vi "calculate.vi"(0 "wm":dbl, 1 "input_1":dbl, 2 "RefpropDirectory":string, 3 "n":i32, 5 "input_2":dbl, 7 "units":enum16{"SI", "IP"}(ring), 9 "InpCode":T1(ring), 11 "error in":errorcluster, 12 "x":dbl[](array[numeric]), 14 "Clear Memory":bool) -> (4 "dataout":dbl[](array[numeric]), 13 "files_path_out":path, 15 "error out":errorcluster)   [LabVIEW 2017]
doc: "Please feel free to contact me if you have any questions .\nMy mail:ken_pop@tom.com yan.ding@jci.com"
panel:
  out "memory counter":i32
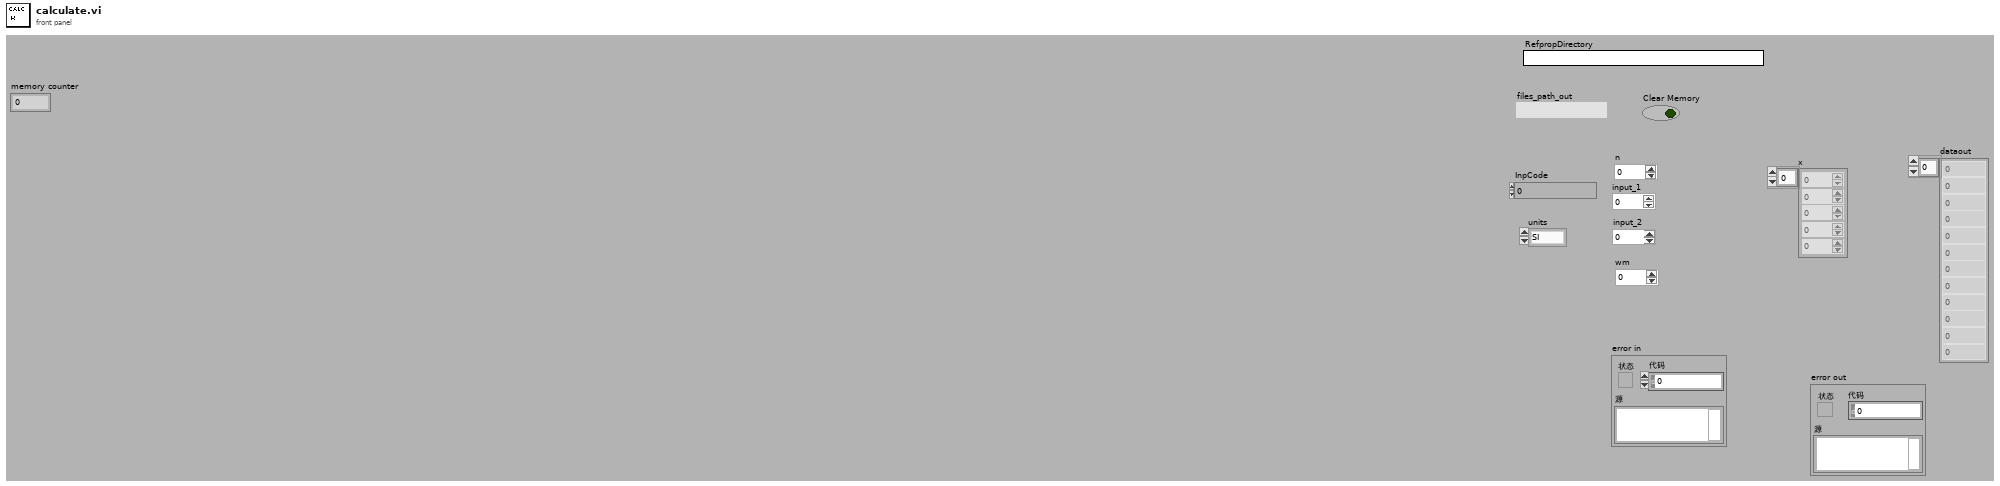
[diagram p1: front panel]
types:
  T1 = enum16{"0", "PS", "HS", "T", "P", "TP", "TH", "TS", "PH", "PQ", "TQ"}
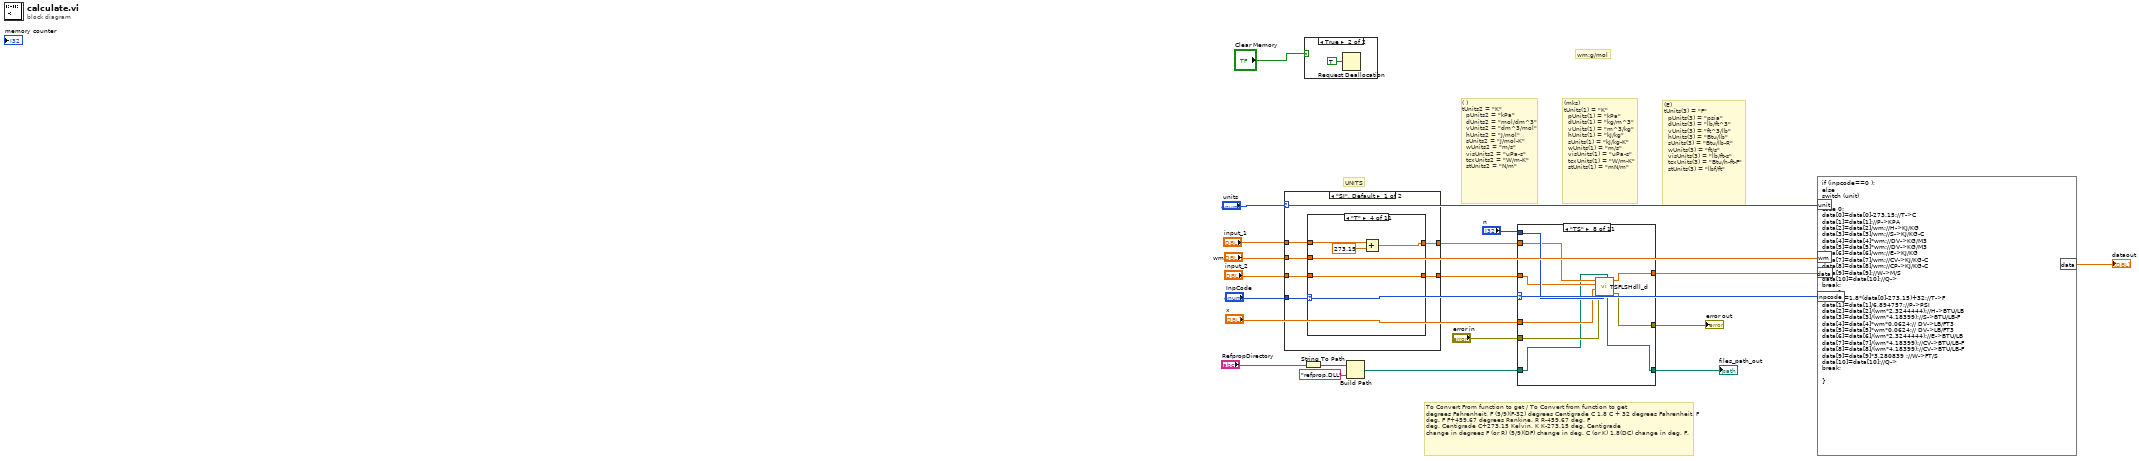
[diagram p0: block diagram]
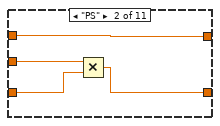
[diagram p4: hidden frame]
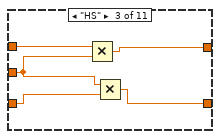
[diagram p5: hidden frame]
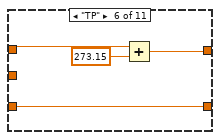
[diagram p7: hidden frame]
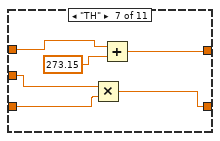
[diagram p8: hidden frame]
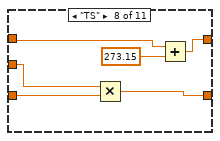
[diagram p9: hidden frame]
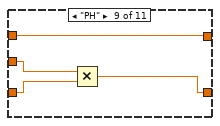
[diagram p10: hidden frame]
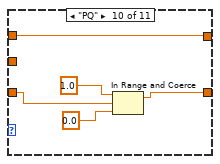
[diagram p11: hidden frame]
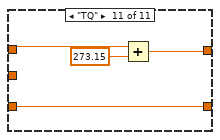
[diagram p12: hidden frame]
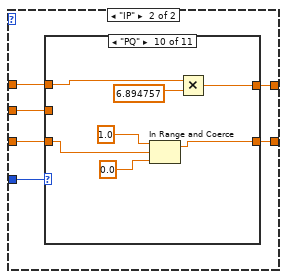
[diagram p13: hidden frame]
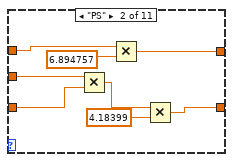
[diagram p15: hidden frame]
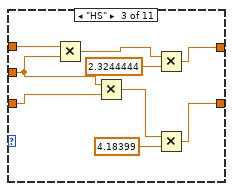
[diagram p16: hidden frame]
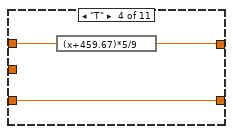
[diagram p17: hidden frame]
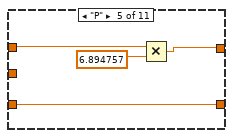
[diagram p18: hidden frame]
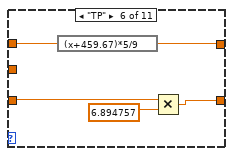
[diagram p19: hidden frame]
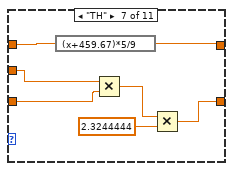
[diagram p20: hidden frame]
diagram:
  # "To Convert From function to get / To Convert from function to get \ndegrees Fahrenheit, F (5/9)(F-32) degrees Centigrade C 1.8 C + 32 degrees Fahrenheit, F \ndeg. F F+459.67 degrees Rankine, R R-459.67 deg. F \ndeg. Centigrade C+273.15 Kelvin, K K-273.15 deg. Centigrade \nchange in degrees F (or R) (5/9)(DF) change in deg. C (or K) 1.8(DC) change in deg. F."
  # "wm:g/mol"
  # "UNITS"
  # "(E)\ntUnits(3) = \"F\"\n  pUnits(3) = \"psia\"\n  dUnits(3) = \"lb/ft^3\"\n  vUnits(3) = \"ft^3/lb\"\n  hUnits(3) = \"Btu/lb\"\n  sUnits(3) = \"Btu/lb-R\"\n  wUnits(3) = \"ft/s\"\n  visUnits(3) = \"lb/ft-s\"\n  tcxUnits(3) = \"Btu/h-ft-F\"\n  stUnits(3) = \"lbf/ft\""
  # "(mks)\ntUnits(1) = \"K\"\n  pUnits(1) = \"kPa\"\n  dUnits(1) = \"kg/m^3\"\n  vUnits(1) = \"m^3/kg\"\n  hUnits(1) = \"kJ/kg\"\n  sUnits(1) = \"kJ/kg-K\"\n  wUnits(1) = \"m/s\"\n  visUnits(1) = \"uPa-s\"\n  tcxUnits(1) = \"W/m-K\"\n  stUnits(1) = \"mN/m\""
  # "( )\ntUnits2 = \"K\"\n  pUnits2 = \"kPa\"\n  dUnits2 = \"mol/dm^3\"\n  vUnits2 = \"dm^3/mol\"\n  hUnits2 = \"J/mol\"\n  sUnits2 = \"J/mol-K\"\n  wUnits2 = \"m/s\"\n  visUnits2 = \"uPa-s\"\n  tcxUnits2 = \"W/m-K\"\n  stUnits2 = \"N/m\""
  n1 = case shown="\"SI\", Default" "units" {
    tunnel: "InpCode" -> [w25 w72]
    tunnel: "input_1" -> [w24 w75]
    tunnel: [w23 w77] -> w9
    tunnel: "input_2" -> [w22 w73]
    tunnel: [w21 w76] -> w7
    tunnel: "wm" -> [w20 w74]
    frame "SI", Default {
      n2 = case shown="\"T\"" w25 {
        tunnel: w24 -> [w27 w31 w36 w39 w42 w45 w51 w57 w59 w65 w70]
        tunnel: [w27 w31 w32 w38 w42 w44 w50 w56 w59 w65 w69] -> w23
        tunnel: w22 -> [w26 w29 w34 w37 w41 w43 w48 w54 w61 w64 w68]
        tunnel: [w26 w28 w33 w37 w41 w43 w47 w53 w60 w63 w68] -> w21
        tunnel: w20 -> [_ w30 w35 _ _ _ w49 w55 w62 _ _]
        frame "0", Default {
        }
        frame "PS" {
          n3 = Multiply(x=w30, y=w29) -> (x*y=w28:dbl)
        }
        frame "HS" {
          n4 = Multiply(x=w36, y=w35) -> (x*y=w32:dbl)
          n5 = Multiply(x=w35, y=w34) -> (x*y=w33:dbl)
        }
        frame "T" {
          n6 = Add(x=w39, y=273.15) -> (x+y=w38:dbl)
        }
        frame "P" {
        }
        frame "TP" {
          n7 = Add(x=w45, y=273.15) -> (x+y=w44:dbl)
        }
        frame "TH" {
          n8 = Multiply(x=w49, y=w48) -> (x*y=w47:dbl)
          n9 = Add(x=w51, y=273.15) -> (x+y=w50:dbl)
        }
        frame "TS" {
          n10 = Multiply(x=w55, y=w54) -> (x*y=w53:dbl)
          n11 = Add(x=w57, y=273.15) -> (x+y=w56:dbl)
        }
        frame "PH" {
          n12 = Multiply(x=w62, y=w61) -> (x*y=w60:dbl)
        }
        frame "PQ" {
          n13 = In Range and Coerce(upper limit=1.0 ("上限"), x=w64, lower limit=0.0 ("下限")) -> (coerced(x)=w63:dbl)  [unwired: 1 out]
        }
        frame "TQ" {
          n14 = Add(x=w70, y=273.15) -> (x+y=w69:dbl)
        }
      }
    }
    frame "IP" {
      n15 = case shown="\"PQ\"" w72 {
        tunnel: w75 -> [w79 w84 w96 w98 w101 w105 w110 w117 w127 w132 w140]
        tunnel: [w79 w83 w88 w97 w100 w104 w109 w116 w126 w131 w139] -> w77
        tunnel: w73 -> [w78 w86 w94 w99 w103 w107 w114 w121 w129 w135 w138]
        tunnel: [w78 w80 w91 w99 w103 w106 w111 w118 w123 w134 w138] -> w76
        tunnel: w74 -> [_ w87 w95 _ _ _ w115 w122 w130 _ _]
        frame "0", Default {
        }
        frame "PS" {
          n16 = Multiply(x=w87, y=w86) -> (x*y=w81:dbl)
          n17 = Multiply(x=w84, y=6.894757) -> (x*y=w83:dbl)
          n18 = Multiply(x=w81, y=4.18399) -> (x*y=w80:dbl)
        }
        frame "HS" {
          n19 = Multiply(x=w96, y=w95) -> (x*y=w89:dbl)
          n20 = Multiply(x=w95, y=w94) -> (x*y=w92:dbl)
          n21 = Multiply(x=w89, y=2.3244444) -> (x*y=w88:dbl)
          n22 = Multiply(x=w92, y=4.18399) -> (x*y=w91:dbl)
        }
        frame "T" {
          n23 = expression code="(x+459.67)*5/9"(w98) -> (w97:dbl)
        }
        frame "P" {
          n24 = Multiply(x=w101, y=6.894757) -> (x*y=w100:dbl)
        }
        frame "TP" {
          n25 = expression code="(x+459.67)*5/9"(w105) -> (w104:dbl)
          n26 = Multiply(x=w107, y=6.894757) -> (x*y=w106:dbl)
        }
        frame "TH" {
          n27 = expression code="(x+459.67)*5/9"(w110) -> (w109:dbl)
          n28 = Multiply(x=w115, y=w114) -> (x*y=w112:dbl)
          n29 = Multiply(x=w112, y=2.3244444) -> (x*y=w111:dbl)
        }
        frame "TS" {
          n30 = expression code="(x+459.67)*5/9"(w117) -> (w116:dbl)
          n31 = Multiply(x=w122, y=w121) -> (x*y=w119:dbl)
          n32 = Multiply(x=w119, y=4.18399) -> (x*y=w118:dbl)
        }
        frame "PH" {
          n33 = Multiply(x=w130, y=w129) -> (x*y=w124:dbl)
          n34 = Multiply(x=w124, y=2.3244444) -> (x*y=w123:dbl)
          n35 = Multiply(x=w127, y=6.894757) -> (x*y=w126:dbl)
        }
        frame "PQ" {
          n36 = In Range and Coerce(upper limit=1.0 ("上限"), x=w135, lower limit=0.0 ("下限")) -> (coerced(x)=w134:dbl)  [unwired: 1 out]
          n37 = Multiply(x=w132, y=6.894757) -> (x*y=w131:dbl)
        }
        frame "TQ" {
          n38 = expression code="(x+459.67)*5/9"(w140) -> (w139:dbl)
        }
      }
    }
  }
  n39 = case shown="True" "Clear Memory" {
    frame False {
    }
    frame True {
      n40 = Request Deallocation(TRUE ("标志")) -> ()
    }
  }
  n41 = String To Path(string="RefpropDirectory") -> (path=w14:path)
  n42 = Build Path(base path=w14, name or relative path="refprop.DLL" ("名称或相对路径")) -> (appended path=w12:path)
  n43 = case shown="\"TS\"" "InpCode" {
    tunnel: "x" -> [_ w154 w159 w169 w176 w184 w193 w201 w210 w217 w223]
    tunnel: "error in" -> [w146 w153 w158 w167 w175 w183 w194 w200 w209 w216 _]
    tunnel: [w146 w152 w162 w166 w174 w182 w195 w199 w208 w215 w225] -> w16
    tunnel: w9 -> [_ w151 w161 w168 w178 w186 w191 w203 w212 w219 w222]
    tunnel: w7 -> [_ w150 w160 _ _ w185 w192 w202 w211 w218 w221]
    tunnel: "n" -> [_ _ _ w170 w177 _ w190 w204 _ _ _]
    tunnel: w12 -> [w145 w149 w157 w164 w173 w180 w189 w198 w207 w220 w227]
    tunnel: [w145 w148 w156 w165 w172 w181 w188 w197 w206 w214 w226] -> w15
    tunnel: [w142 w147 w155 w163 w171 w179 w187 w196 w205 w213 w224] -> w6
    frame "0", Default {
      n44 = Initialize Array(0.0 ("元素"), 10 ("维数大小")) -> (w142:dbl[])
    }
    frame "PS" {
      n45 = call "PSFLSHdll_d.vi"("dll_path_in"=w149, "error in (no error)"=w153, "Component Molar Fractions"=w154, "p"=w151, "S"=w150) -> ("error out"=w152:errorcluster, "psdataout"=w147:dbl[], "dll_path_out"=w148:path)  [unwired: 4 in]
    }
    frame "HS" {
      n46 = call "HSFLSHdll_d.vi"("dll_path_in"=w157, "error in (no error)"=w158, "Component Molar Fractions"=w159, "H"=w161, "S"=w160) -> ("error out"=w162:errorcluster, "HSdataout"=w155:dbl[], "dll_path_out"=w156:path)  [unwired: 4 in]
    }
    frame "T" {
      n47 = call "SATTdll_d.vi"("Refpropdllpath"=w164, "error in (no error)"=w167, "Component Molar Fractions"=w169, "i"=w170, "Temp (deg C)"=w168) -> ("error out"=w166:errorcluster, "tdataout"=w163:dbl[], "dll_path_out"=w165:path)  [unwired: 4 in]
    }
    frame "P" {
      n48 = call "SATPdll_d.vi"("dll_path_in"=w173, "error in (no error)"=w175, "Component Molar Fractions"=w176, "i"=w177, "Press (kPa)"=w178) -> ("error out"=w174:errorcluster, "pdataout"=w171:dbl[], "dll_path_out"=w172:path)  [unwired: 4 in]
    }
    frame "TP" {
      n49 = call "TPFLSHdll_d.vi"("dll_path_in"=w180, "error in (no error)"=w183, "Component Molar Fractions"=w184, "p"=w185, "Temp (deg c)"=w186) -> ("error out"=w182:errorcluster, "TPDATAOUT"=w179:dbl[], "dll_path_out"=w181:path)  [unwired: 4 in]
    }
    frame "TH" {
      n50 = call "THFLSHdll_d.vi"("dll_path_in"=w189, "i"=w190, "error in (no error)"=w194, "Component Molar Fractions"=w193, "h"=w192, "Temp (deg c)"=w191) -> ("error out"=w195:errorcluster, "THDATAOUT"=w187:dbl[], "dll_path_out"=w188:path)  [unwired: 3 in]
    }
    frame "TS" {
      n51 = call "TSFLSHdll_d.vi"("dll_path_in"=w198, "i"=w204, "error in (no error)"=w200, "Component Molar Fractions"=w201, "S"=w202, "Temp (deg c)"=w203) -> ("error out"=w199:errorcluster, "TSDATAOUT"=w196:dbl[], "dll_path_out"=w197:path)  [unwired: 3 in]
    }
    frame "PH" {
      n52 = call "PHFLSHdll_d.vi"("dll_path_in"=w207, "error in (no error)"=w209, "Component Molar Fractions"=w210, "H"=w211, "P"=w212) -> ("error out"=w208:errorcluster, "phdataout"=w205:dbl[], "dll_path_out"=w206:path)  [unwired: 4 in]
    }
    frame "PQ" {
      n53 = call "PQFLSHdll_d.vi"("dll_path_in"=w220, "error in (no error)"=w216, "Component Molar Fractions"=w217, "Q"=w218, "P"=w219) -> ("error out"=w215:errorcluster, "pqdataout"=w213:dbl[], "dll_path_out"=w214:path)  [unwired: 4 in]
    }
    frame "TQ" {
      n54 = call "TQFLSHdll_d.vi"("dll_path_in"=w227, "Component Molar Fractions"=w223, "Q"=w221, "T"=w222) -> ("error out"=w225:errorcluster, "tqdataout"=w224:dbl[], "dll_path_out"=w226:path)  [unwired: 5 in]
    }
  }
  "error out" <- w16
  "files_path_out" <- w15
  n55 = formula code="if (inpcode==0 );\nelse\nswitch (unit)\n{\ncase 0:\ndata[0]=data[0]-273.15;//T->C\ndata[1]=data[1];//P->KPA\ndata[2]=data[2]/wm;//H->KJ/KG\ndata[3]=data[3]/wm;//S->KJ/KG-C\ndata[4]=data[4]*wm;//DV->KG/M3\ndata[5]=data[5]*wm;//DV->KG/M3\ndata[6]=data[6]/wm;//E->KJ/KG\ndata[7]=data[7]/wm;//CV->KJ/KG-C\ndata[8]=data[8]/wm;//CP->KJ/KG-C\ndata[9]=data[9];//W->M/S\ndata[10]=data[10];//Q->\nbreak;\ncase 1:\ndata[0]=1.8*(data[0]-273.15)+32;//T->F\ndata[1]=data[1]/6.894757;//P->PSI\ndata[2]=data[2]/(wm*2.3244444);//H->BTU/LB\ndata[3]=data[3]/(wm*4.18399);//S->BTU/LB-F\ndata[4]=data[4]*wm*0.0624;// DV->LB/FT3\ndata[5]=data[5]*wm*0.0624;// DV->LB/FT3\ndata[6]=data[6]/(wm*2.3244444);//E->BTU/LB\ndata[7]=data[7]/(wm*4.18399);//CV->BTU/LB-F\ndata[8]=data[8]/(wm*4.18399);//CV->BTU/LB-F\ndata[9]=data[9]*3.280839 ;//W->FT/S\ndata[10]=data[10];//Q->\nbreak;\n\n}"("data"=w6, "unit"="units", "inpcode"="InpCode", "wm"="wm") -> ("data"=→"dataout":dbl[])
